vi "ScanInfo.vi"(0 "refnum":refnum<file>, 11 "offset":i32) -> (2 "Scan Info":T1 {"delay" format="%.2f"; "pivot distance" format="%.2f"; "sector scan angle" format="%.2f"}, 4 "dup refnum":refnum<file>, 6 "delay":sgl format="%.2f", 8 "pivot distance":sgl format="%.2f", 10 "sector scan angle":sgl format="%.2f", 13 "location":string, 14 "Scan Mode":string, 15 "operator":string)   [LabVIEW 2022 SP3]
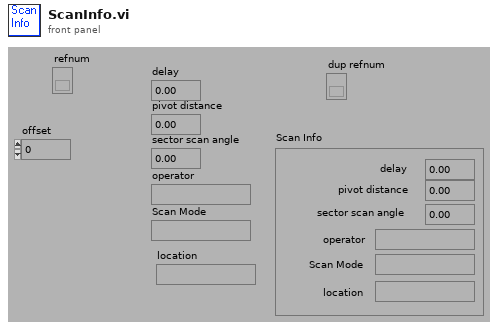
[diagram p1: front panel]
types:
  T1 = cluster{"delay":sgl, "pivot distance":sgl, "sector scan angle":sgl, "operator":string, "Scan Mode":string, "location":string}
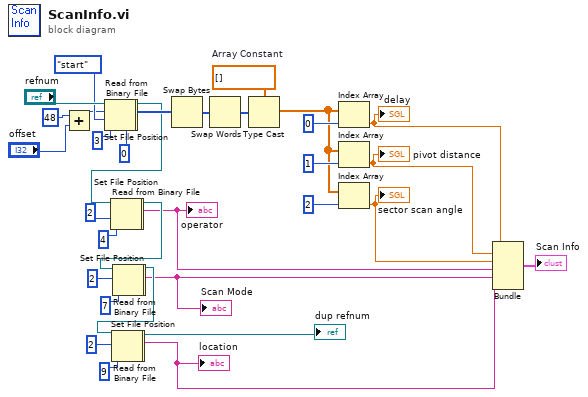
[diagram p0: block diagram]
diagram:
  w33 = sgl[] []  # Array Constant
  n1 = Add(x=48 ("pos offset (0)"), y="offset") -> (x+y=w10:i32)
  n2 = Set File Position(offset (in bytes) (0)=w10, refnum="refnum", from (0:start)=enum16{"start", "end", "current"}."start" ("pos mode (0:2)")) -> (refnum out=w2:refnum<file>, error out=w1:errorcluster)  [unwired: 1 in]
  n3 = Read from Binary File(5:0 ("byte stream type"), 8:w1, 10:3 ("count"), 11:w2) -> (2:w35:i32[], 3:w26:refnum<file>)  [unwired: 4 out]
  n4 = Set File Position(refnum=w26, from (0:start)=2) -> (refnum out=w4:refnum<file>, error out=w3:errorcluster)  [unwired: 1 in, 1 out]
  n5 = Read from Binary File(8:w3, 10:4 ("count"), 11:w4) -> (2:w15:string, 3:w23:refnum<file>)  [unwired: 5 out]
  "operator" <- w15
  n6 = Set File Position(refnum=w23, from (0:start)=2) -> (refnum out=w6:refnum<file>, error out=w5:errorcluster)  [unwired: 1 in, 1 out]
  n7 = Read from Binary File(8:w5, 10:7 ("count"), 11:w6) -> (2:w14:string, 3:w20:refnum<file>)  [unwired: 5 out]
  "Scan Mode" <- w14
  n8 = Set File Position(refnum=w20, from (0:start)=2) -> (refnum out=w8:refnum<file>, error out=w7:errorcluster)  [unwired: 1 in, 1 out]
  n9 = Read from Binary File(8:w7, 10:9 ("count"), 11:w8) -> (2:w13:string, 3:→"dup refnum":refnum<file>)  [unwired: 5 out]
  "location" <- w13
  n10 = Swap Bytes(anything=w35) -> (byte swapped=w34:i32[])
  n11 = Swap Words(1:w34) -> (0:w32:i32[])
  n12 = Type Cast(type=w33, x=w32) -> (*(type *) &x=w31:sgl[])
  n13 = Index Array(array=w31, index=0) -> (element=w18:sgl)
  "delay" <- w18
  n14 = Index Array(array=w31, index=1) -> (element=w17:sgl)
  "pivot distance" <- w17
  n15 = Index Array(array=w31, index=2) -> (element=w16:sgl)
  "sector scan angle" <- w16
  n16 = Bundle(w18, w17, w16, w15, w14, w13) -> (→"Scan Info":cluster{sgl, sgl, sgl, string, string, string})  [unwired: 1 out]
